vi "Get Engine Trigger State.vi"(10 "Bus State":T1, 11 "Log in":bool) -> (2 "Log Trigger":bool, 3 "Log out":bool)   [LabVIEW 2019, in "CAN Stream Support Workspace Shared.lvlib"]
uses:
  CAN Stream Support Workspace Shared.lvlib
  Types/Host Stream Engine State.ctl
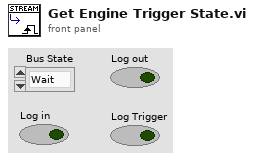
[diagram p1: front panel]
types:
  T1 = typedef "CAN Stream Support Workspace Shared.lvlib/Host Stream Engine State.ctl" = enum8{"Wait", "Start Stream", "Read Stream", "Stop Stream", "Exit"}
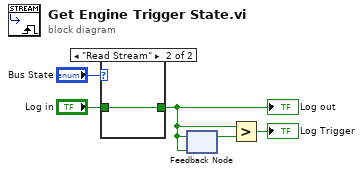
[diagram p0: block diagram]
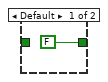
[diagram p2: hidden frame]
diagram:
  n1 = case shown="\"Read Stream\"" "Bus State" {
    tunnel: [FALSE ("Log") w7] -> w3
    tunnel: "Log in" -> [_ w7]
    frame Default {
    }
    frame "Read Stream" {
    }
  }
  "Log out" <- w3
  n2 = feedback #1(w3) -> (w1:bool)
  n3 = feedback-in #1(w3) -> ()
  n4 = Greater?(x=w3, y=w1) -> (0:→"Log Trigger":bool)
